vi "Set_Build_Data.vi"(8 "error in (no error)":errorcluster, 10 "data":T1, 11 "Class in":refnum<class "AB_Build.lvclass">) -> (0 "error out":errorcluster, 3 "Class out":refnum<class "AB_Build.lvclass">)   [LabVIEW 2020, in "AB_Build.lvclass"]
uses:
  <vilib>/AppBuilder/AB_Classes/Build/AB_Build.lvclass
  <vilib>/AppBuilder/AB_Classes/Build/AB_Build.ctl
  <vilib>/AppBuilder/AB_Classes/PreviewCache/PreviewCache.lvclass
  <vilib>/AppBuilder/AB_Classes/Destination/AB_Destination.lvclass
  <vilib>/AppBuilder/AB_Exclusion_Option.ctl
  <resource>/Framework/Providers/API/ItemRef.ctl
  <resource>/Framework/Providers/Common/provcom_ProgressBar_Events.ctl
  <resource>/Framework/Providers/API/mxLvBuildError.ctl
  <vilib>/AppBuilder/AB_Classes/Build/AB_Build.lvclass/AB_Build.ctl
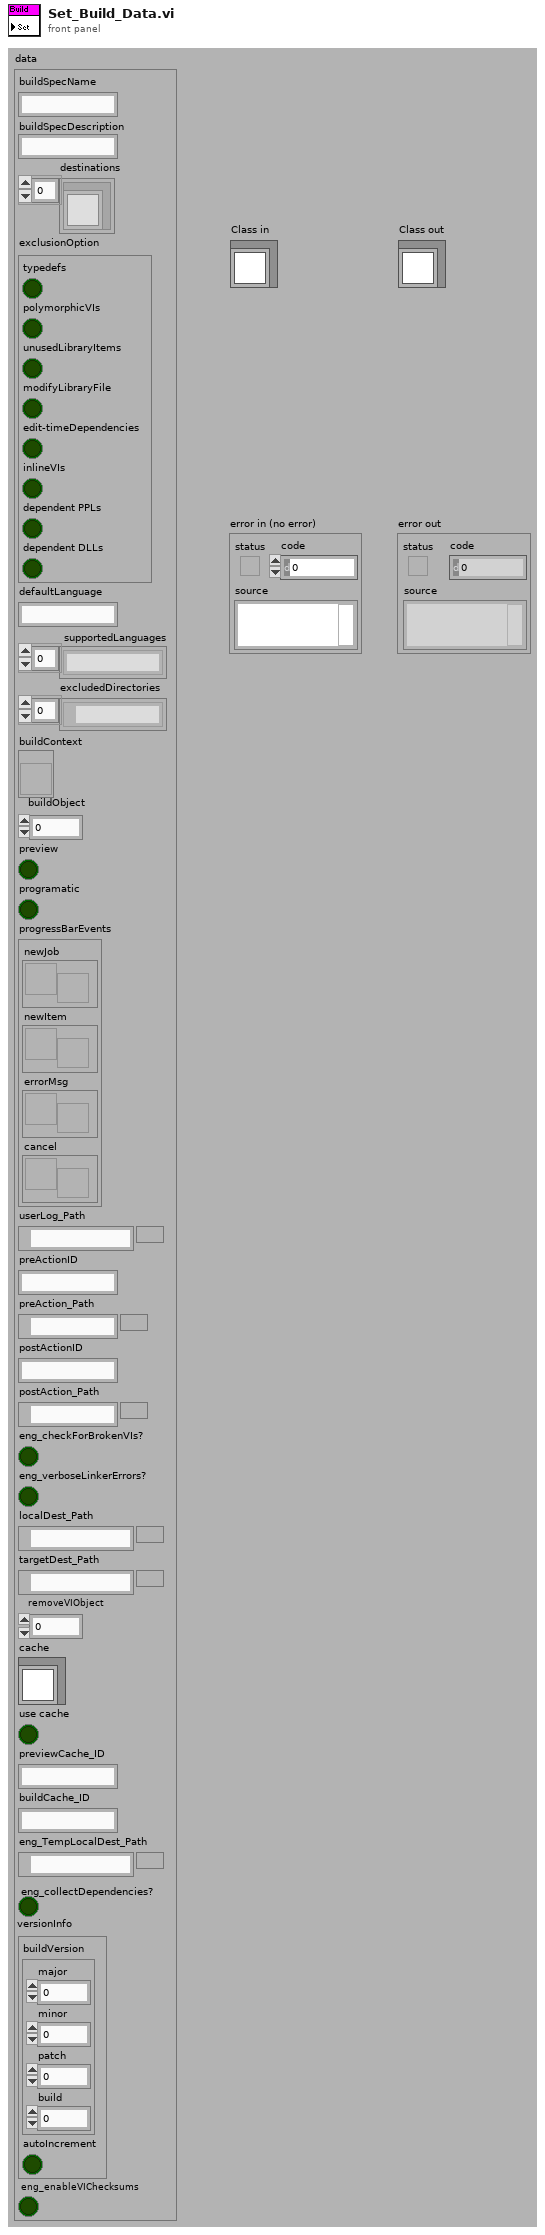
[diagram p1: front panel]
types:
  T1 = typedef "AB_Build.ctl" = cluster{"buildSpecName":string, "buildSpecDescription":string, "destinations":refnum<class "AB_Destination.lvclass">[], "exclusionOption":T2, "defaultLanguage":string, "supportedLanguages":string[], "excludedDirectories":path[], "buildContext":refnum<vi>, "buildObject":T3, "preview":bool, "programatic":bool, "progressBarEvents":T4, "userLog_Path":path, "preActionID":string, "preAction_Path":path, "postActionID":string, "postAction_Path":path, "eng_checkForBrokenVIs?":bool, "eng_verboseLinkerErrors?":bool, "localDest_Path":path, "targetDest_Path":path, "removeVIObject":u16, "cache":refnum<class "PreviewCache.lvclass">, "use cache":bool, "previewCache_ID":string, "buildCache_ID":string, "eng_TempLocalDest_Path":path, "eng_collectDependencies?":bool, "versionInfo":cluster{"buildVersion":cluster{"major":u16, "minor":u16, "patch":u16, "build":u16}, "autoIncrement":bool}, "eng_enableVIChecksums":bool}
  T2 = typedef "AB_Exclusion_Option.ctl" = cluster{"typedefs":bool, "polymorphicVIs":bool, "unusedLibraryItems":bool, "modifyLibraryFile":bool, "edit-timeDependencies":bool, "inlineVIs":bool, "dependent PPLs":bool, "dependent DLLs":bool}
  T3 = typedef "ItemRef.ctl" = u64
  T4 = typedef "provcom_ProgressBar_Events.ctl" = cluster{"newJob":refnum<user-event>, "newItem":refnum<user-event>, "errorMsg":T5, "cancel":refnum<user-event>}
  T5 = typedef "mxLvBuildError.ctl" = refnum<user-event>
  T6 = cluster{"buildVersion":cluster{"major":u16, "minor":u16, "patch":u16, "build":u16}, "autoIncrement":bool}
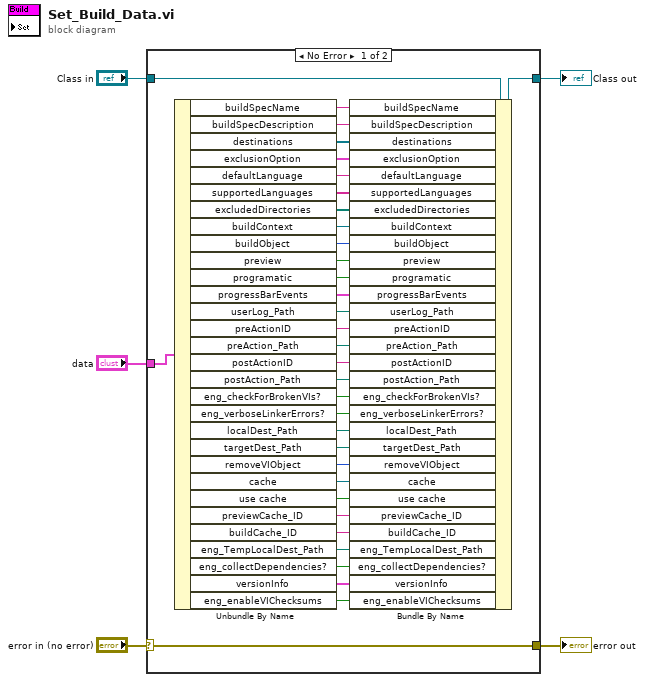
[diagram p0: block diagram]
diagram:
  n1 = case "Case" shown="No Error" "error in (no error)" {
    selector: "error in (no error)" -> [w39 w41]
    tunnel: [w39 w41] -> w4
    tunnel: [w38 w40] -> w2
    tunnel: "Class in" -> [w37 w40]
    tunnel: "data" -> [w36 _]
    frame No Error {
      n2 = Unbundle By Name(w36) -> ("buildSpecName"=w27:string, "buildSpecDescription"=w24:string, "destinations"=w35:refnum<class "AB_Destination.lvclass">[], "exclusionOption"=w34:T2, "defaultLanguage"=w33:string, "supportedLanguages"=w32:string[], "excludedDirectories"=w31:path[], "buildContext"=w30:refnum<vi>, "buildObject"=w29:T3, "preview"=w28:bool, "programatic"=w26:bool, "progressBarEvents"=w25:T4, "userLog_Path"=w23:path, "preActionID"=w22:string, "preAction_Path"=w21:path, "postActionID"=w20:string, "postAction_Path"=w19:path, "eng_checkForBrokenVIs?"=w18:bool, "eng_verboseLinkerErrors?"=w17:bool, "localDest_Path"=w16:path, "targetDest_Path"=w15:path, "removeVIObject"=w14:u16, "cache"=w13:refnum<class "PreviewCache.lvclass">, "use cache"=w12:bool, "previewCache_ID"=w11:string, "buildCache_ID"=w9:string, "eng_TempLocalDest_Path"=w10:path, "eng_collectDependencies?"=w8:bool, "versionInfo"=w7:T6, "eng_enableVIChecksums"=w6:bool)
      n3 = Bundle By Name(cluster=w37, "buildSpecName"=w27, "buildSpecDescription"=w24, "destinations"=w35, "exclusionOption"=w34, "defaultLanguage"=w33, "supportedLanguages"=w32, "excludedDirectories"=w31, "buildContext"=w30, "buildObject"=w29, "preview"=w28, "programatic"=w26, "progressBarEvents"=w25, "userLog_Path"=w23, "preActionID"=w22, "preAction_Path"=w21, "postActionID"=w20, "postAction_Path"=w19, "eng_checkForBrokenVIs?"=w18, "eng_verboseLinkerErrors?"=w17, "localDest_Path"=w16, "targetDest_Path"=w15, "removeVIObject"=w14, "cache"=w13, "use cache"=w12, "previewCache_ID"=w11, "buildCache_ID"=w9, "eng_TempLocalDest_Path"=w10, "eng_collectDependencies?"=w8, "versionInfo"=w7, "eng_enableVIChecksums"=w6) -> (w38:refnum<class "AB_Build.lvclass">)
    }
    frame Error {
    }
  }
  "error out" <- w4
  "Class out" <- w2
